vi "calc_phase_map.vi"(3 "noise threshold":dbl=20.0, 4 "u8_ar_image_pixel_array":dbl[][][](array[numeric]), 5 "image name":string="fringe") -> (0 "raw phase map array":u8[][](array[numeric]), 1 "u8_ar_noise_mask":u8[][](array[numeric]), 2 "phase map":T1(plugin-control))   [LabVIEW 2011]
uses:
  global_vars.vi
panel:
  in  "add":dbl
  in  "multi":dbl
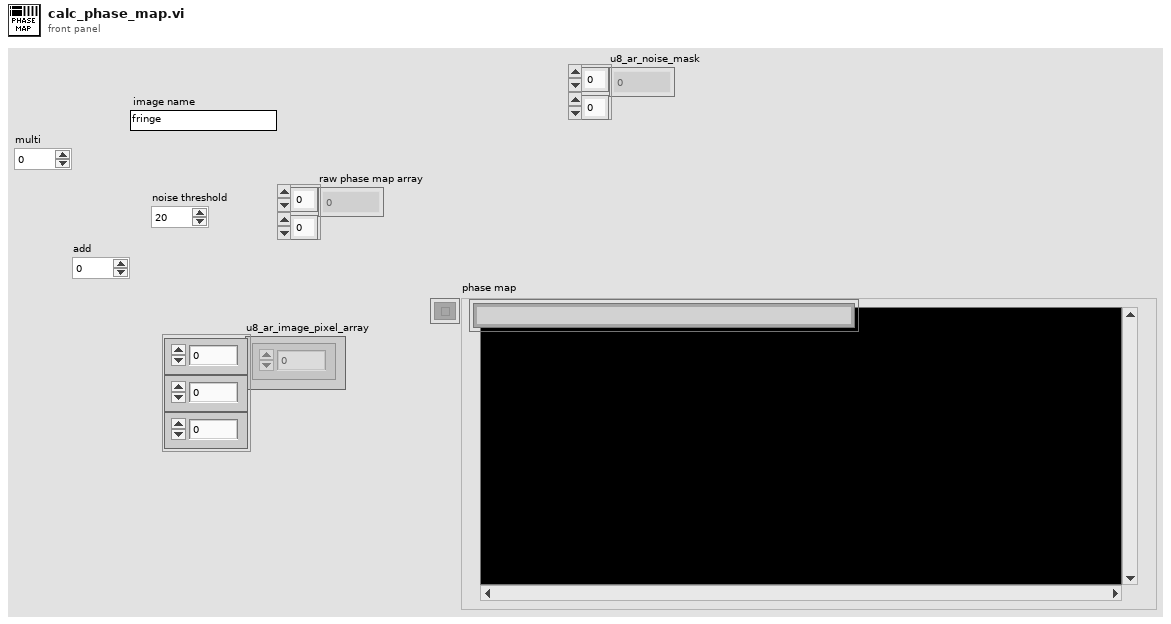
[diagram p1: front panel]
types:
  T1 = typedef "IMAQ Image.ctl" = refnum<image>
  T2 = typedef "Image Type" = u32
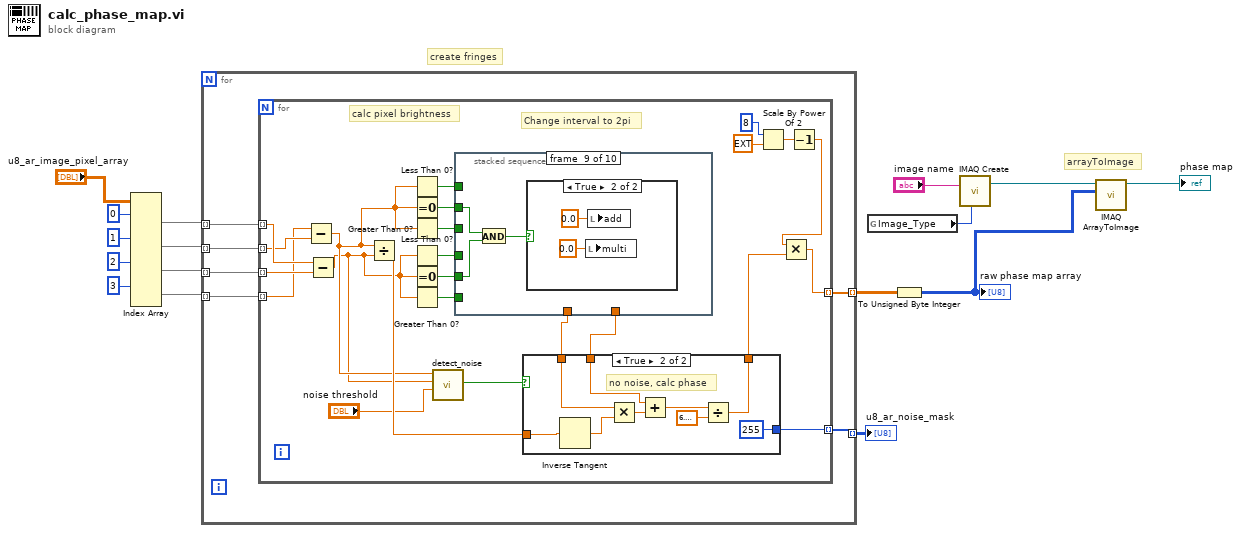
[diagram p0: block diagram]
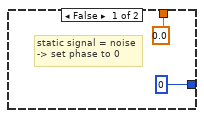
[diagram p2: hidden frame]
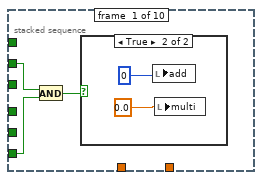
[diagram p3: hidden frame]
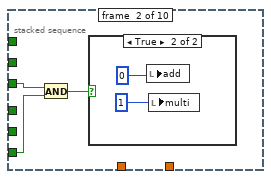
[diagram p5: hidden frame]
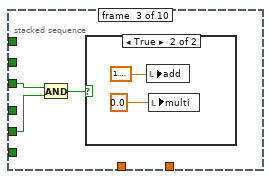
[diagram p7: hidden frame]
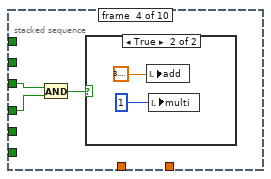
[diagram p9: hidden frame]
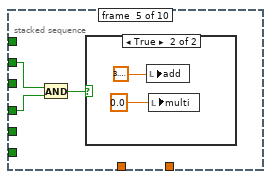
[diagram p11: hidden frame]
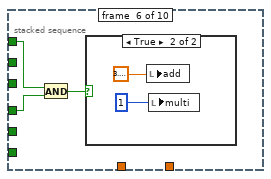
[diagram p13: hidden frame]
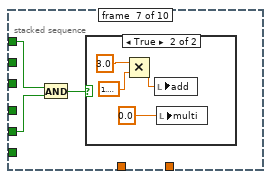
[diagram p15: hidden frame]
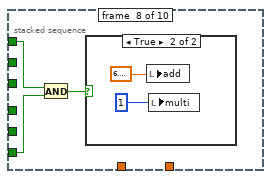
[diagram p17: hidden frame]
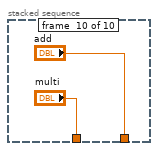
[diagram p20: hidden frame]
diagram:
  # "arrayToImage"
  # "create fringes"
  n1 = Index Array(array="u8_ar_image_pixel_array", index (dim 0) #1=0 ("index (page)"), index (dim 0) #2=1 ("index (page)"), index (dim 0) #3=2 ("index (page)"), index (dim 0) #4=3 ("index (page)")) -> (element #1=w12:dbl[][], element #2=w11:dbl[][], element #3=w10:dbl[][], element #4=w9:dbl[][])  [unwired: 8 in]
  n2 = for {
    tunnel: w12 -> [w22] mode=indexing
    tunnel: w11 -> [w21] mode=indexing
    tunnel: w10 -> [w20] mode=indexing
    tunnel: w9 -> [w19] mode=indexing
    tunnel: [w18] -> w8 mode=indexing
    tunnel: [w17] -> w1 mode=indexing
    n3 = for {
      tunnel: w22 -> [w34] mode=indexing
      tunnel: w21 -> [w33] mode=indexing
      tunnel: w20 -> [w30] mode=indexing
      tunnel: w19 -> [w29] mode=indexing
      tunnel: [w42] -> w18 mode=indexing
      tunnel: [w23] -> w17 mode=indexing
      # "Change interval to 2pi"
      # "calc pixel brightness"
      n4 = Subtract(x=w29, y=w33) -> (x-y=w26:dbl)
      n5 = Subtract(x=w34, y=w30) -> (x-y=w25:dbl)
      n6 = Divide(x=w26, y=w25) -> (x/y=w28:dbl)
      n7 = Less Than 0?(x=w26) -> (x < 0?=w40:bool)
      n8 = Equal To 0?(x=w26) -> (x = 0?=w39:bool)
      n9 = Greater Than 0?(x=w26) -> (x > 0?=w38:bool)
      n10 = Less Than 0?(x=w25) -> (x < 0?=w35:bool)
      n11 = Equal To 0?(x=w25) -> (x = 0?=w36:bool)
      n12 = Greater Than 0?(x=w25) -> (x > 0?=w37:bool)
      n13 = call "detect_noise.vi"("threshold"="noise threshold", "i1-i3"=w25, "i4-i2"=w26) -> ("is signal"=w27:bool)  [unwired: 8 in]
      n14 = stacked-sequence {
        tunnel: w40 -> [_ _ _ _ _ w84 w89 w95 _ _]
        tunnel: w39 -> [w59 _ _ _ w79 _ _ _ w100 _]
        tunnel: w38 -> [_ w64 w68 w74 _ _ _ _ _ _]
        tunnel: w37 -> [w58 w63 _ _ _ _ _ w96 _ _]
        tunnel: w36 -> [_ _ w69 _ _ _ w88 _ w101 _]
        tunnel: w35 -> [_ _ _ w73 w78 w83 _ _ _ _]
        tunnel: [_ _ _ _ _ _ _ _ _ "add"] -> w32
        tunnel: [_ _ _ _ _ _ _ _ _ "multi"] -> w31
        frame #0 {
          n15 = And(x=w59, y=w58) -> (x .and. y?=w60:bool)
          n16 = case shown="True" w60 {
            frame False {
            }
            frame True {
              n17 = local write "add"(0) -> ()
              n18 = local write "multi"(0.0) -> ()
            }
          }
        }
        frame #1 {
          n19 = And(x=w64, y=w63) -> (x .and. y?=w65:bool)
          n20 = case shown="True" w65 {
            frame False {
            }
            frame True {
              n21 = local write "add"(0) -> ()
              n22 = local write "multi"(1) -> ()
            }
          }
        }
        frame #2 {
          n23 = And(x=w68, y=w69) -> (x .and. y?=w70:bool)
          n24 = case shown="True" w70 {
            frame False {
            }
            frame True {
              n25 = local write "add"(1.5707963267948966) -> ()
              n26 = local write "multi"(0.0) -> ()
            }
          }
        }
        frame #3 {
          n27 = And(x=w74, y=w73) -> (x .and. y?=w75:bool)
          n28 = case shown="True" w75 {
            frame False {
            }
            frame True {
              n29 = local write "add"(3.141592653589793) -> ()
              n30 = local write "multi"(1) -> ()
            }
          }
        }
        frame #4 {
          n31 = And(x=w79, y=w78) -> (x .and. y?=w80:bool)
          n32 = case shown="True" w80 {
            frame False {
            }
            frame True {
              n33 = local write "add"(3.141592653589793) -> ()
              n34 = local write "multi"(0.0) -> ()
            }
          }
        }
        frame #5 {
          n35 = And(x=w84, y=w83) -> (x .and. y?=w85:bool)
          n36 = case shown="True" w85 {
            frame False {
            }
            frame True {
              n37 = local write "add"(3.141592653589793) -> ()
              n38 = local write "multi"(1) -> ()
            }
          }
        }
        frame #6 {
          n39 = And(x=w89, y=w88) -> (x .and. y?=w90:bool)
          n40 = case shown="True" w90 {
            frame False {
            }
            frame True {
              n41 = Multiply(x=3.0, y=1.5707963267948966) -> (x*y=w93:dbl)
              n42 = local write "add"(w93) -> ()
              n43 = local write "multi"(0.0) -> ()
            }
          }
        }
        frame #7 {
          n44 = And(x=w95, y=w96) -> (x .and. y?=w97:bool)
          n45 = case shown="True" w97 {
            frame False {
            }
            frame True {
              n46 = local write "add"(6.283185307179586) -> ()
              n47 = local write "multi"(1) -> ()
            }
          }
        }
        frame #8 {
          n48 = And(x=w100, y=w101) -> (x .and. y?=w102:bool)
          n49 = case shown="True" w102 {
            frame False {
            }
            frame True {
              n50 = local write "multi"(0.0 ("multi")) -> ()
              n51 = local write "add"(0.0 ("add")) -> ()
            }
          }
        }
        frame #9 {
        }
      }
      n52 = case shown="True" w27 {
        tunnel: [0.0 w51] -> w43
        tunnel: w32 -> [_ w50]
        tunnel: w31 -> [_ w54]
        tunnel: w28 -> [_ w53]
        tunnel: [u8 0 u8 255] -> w23
        frame False {
          # "static signal = noise\n-> set phase to 0"
        }
        frame True {
          # "no noise, calc phase"
          n53 = Inverse Tangent(1:w53) -> (0:w52:dbl)
          n54 = Multiply(x=w54, y=w52) -> (x*y=w55:dbl)
          n55 = Add(x=w50, y=w55) -> (x+y=w56:dbl)
          n56 = Divide(x=w56, y=6.283185307179586) -> (x/y=w51:dbl)
        }
      }
      n57 = Scale By Power Of 2(n=8, x=ext 1.0) -> (x*2^n=w45:ext)
      n58 = Decrement(x=w45) -> (x-1=w44:ext)
      n59 = Multiply(x=w44, y=w43) -> (x*y=w42:ext)
    }
  }
  "u8_ar_noise_mask" <- w1
  n60 = global read "global_vars.vi" "Image_Type"() -> (w3:T2)
  n61 = To Unsigned Byte Integer(number=w8) -> (unsigned 8bit integer=w2:u8[][])
  "raw phase map array" <- w2
  n62 = call "IMAQ Create"("Image Name"="image name", "Image Type"=w3) -> ("New Image"=w4:T1)  [unwired: 2 in, 2 out]
  n63 = call "IMAQ ArrayToImage"("Image Pixels (U8)"=w2, "Image"=w4) -> ("Image Out"=→"phase map":T1)  [unwired: 8 in, 1 out]
